vi "Release All Notifiers.vi"(8 "error in (no error)":errorcluster, 11 "All Data Notifiers":T1) -> (0 "error out":errorcluster)   [LabVIEW 2013, in "Data Notifiers.lvlib"]
uses:
  Data Notifiers.lvlib
  All Data Notifiers.ctl
  Acquisition/APD Notifier Cluster.ctl
  Piezo/Piezo display.ctl
  XY/XY Display.ctl
  Capacitive/Capacitive Signal Cluster.ctl
  Feedback/Control 2.ctl
  Acquisition/Acquisition.lvlib
  Piezo/Piezo.lvlib
  XY/XY.lvlib
  Capacitive/Capacitive.lvlib
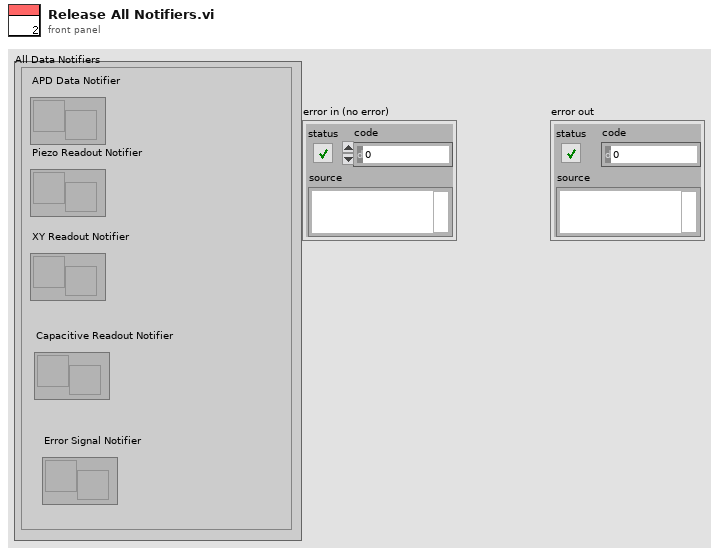
[diagram p1: front panel]
types:
  T1 = typedef "Data Notifiers.lvlib/All Data Notifiers.ctl" = cluster{"APD Data Notifier":refnum<notifier>, "Piezo Readout Notifier":refnum<notifier>, "XY Readout Notifier":refnum<notifier>, "Capacitive Readout Notifier":refnum<notifier>, "Error Signal Notifier":refnum<notifier>}
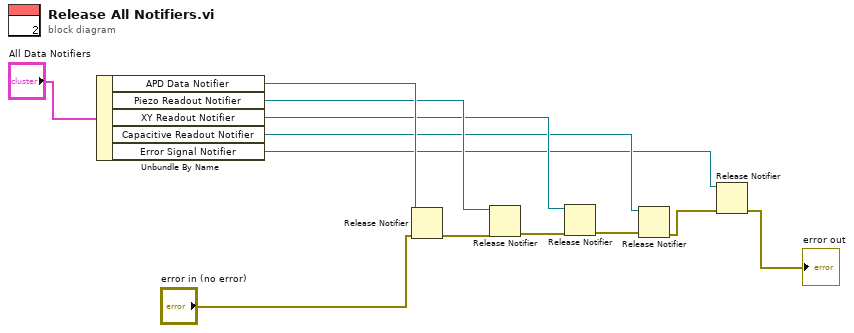
[diagram p0: block diagram]
diagram:
  n1 = Unbundle By Name("All Data Notifiers") -> ("APD Data Notifier"=w11:refnum<notifier>, "Piezo Readout Notifier"=w10:refnum<notifier>, "XY Readout Notifier"=w9:refnum<notifier>, "Capacitive Readout Notifier"=w8:refnum<notifier>, "Error Signal Notifier"=w1:refnum<notifier>)
  n2 = Release Notifier(notifier=w11, error in (no error)="error in (no error)") -> (error out=w7:errorcluster)  [unwired: 1 in, 2 out]
  n3 = Release Notifier(notifier=w10, error in (no error)=w7) -> (error out=w6:errorcluster)  [unwired: 1 in, 2 out]
  n4 = Release Notifier(notifier=w9, error in (no error)=w6) -> (error out=w5:errorcluster)  [unwired: 1 in, 2 out]
  n5 = Release Notifier(notifier=w8, error in (no error)=w5) -> (error out=w3:errorcluster)  [unwired: 1 in, 2 out]
  n6 = Release Notifier(notifier=w1, error in (no error)=w3) -> (error out=→"error out":errorcluster)  [unwired: 1 in, 2 out]
